vi "PicoScope5000aGetRapidBlockBulk.vi"(0 "error in":errorcluster, 5 "Device Info":T2, 7 "handle in":i16, 9 "enabled array":i16[](array[numeric]), 11 "Rapid Block Acquisition Settings":T1={"preTriggerSamples"=0, "postTriggerSamples"=1000, "timebase"=2, "Down-Sample Mode"=0, "Down Sample Ratio"=1, "Number of Captures"=10} {"Down Sample Ratio" min=1 step=1; "Down-Sample Mode" items=["None"=0, "Aggregate"=1, "Decimate"=2, "Average"=4]}) -> (2 "Channel A Buffer":i16[][](array[numeric]), 3 "Channel B Buffer":i16[][](array[numeric]), 4 "error out":errorcluster, 6 "handle out":i16, 8 "Port 0":i16[][](array[numeric]), 10 "Port 1":i16[][](array[numeric]), 12 "Num samples":u32, 13 "Channel C Buffer":i16[][](array[numeric]), 14 "Channel D Buffer":i16[][](array[numeric]))   [LabVIEW 2020]
doc: "This VI gets a set of blocks captured using rapid block mode. It outputs two-dimensional arrays for each channel that contain data from all the requested captures."
uses:
  ps5000a.dll
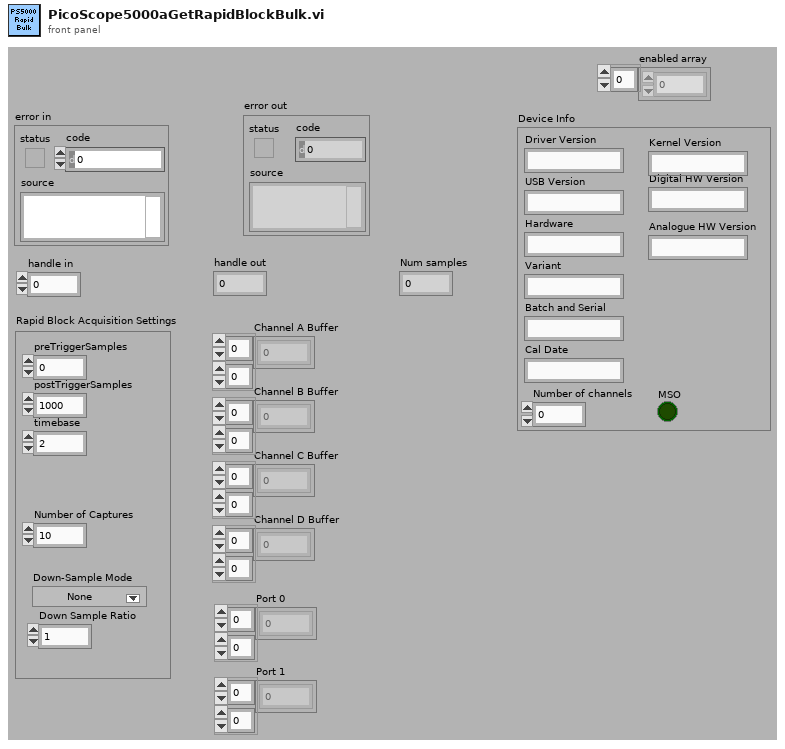
[diagram p1: front panel]
types:
  T1 = cluster{"preTriggerSamples":u32, "postTriggerSamples":u32, "timebase":u32, "Down-Sample Mode":i32, "Down Sample Ratio":u32, "Number of Captures":u32}
  T2 = cluster{"Driver Version":string, "USB Version":string, "Hardware":string, "Variant":string, "Batch and Serial":string, "Cal Date":string, "Kernel Version":string, "Digital HW Version":string, "Analogue HW Version":string, "MSO":bool, "Number of channels":i16}
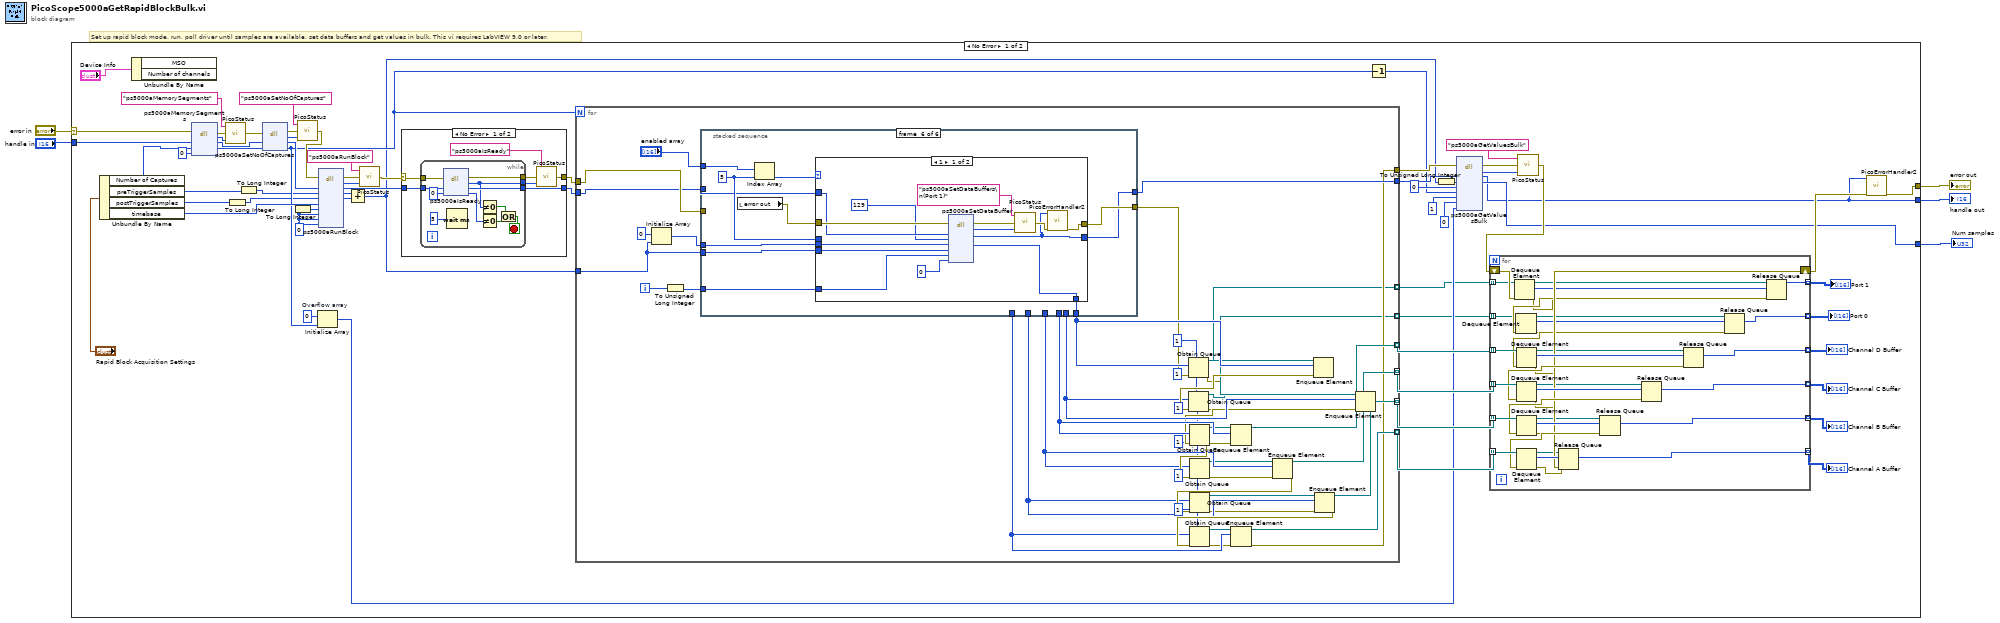
[diagram p0: block diagram]
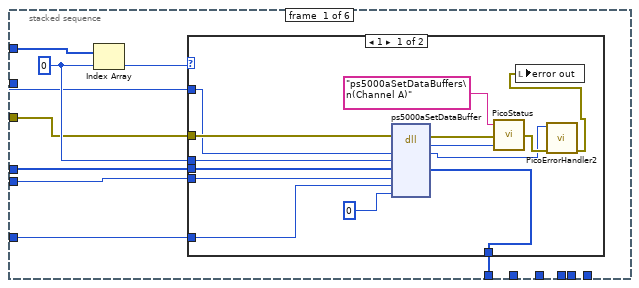
[diagram p2: hidden frame]
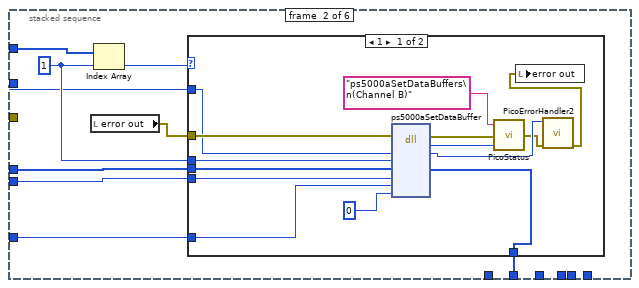
[diagram p4: hidden frame]
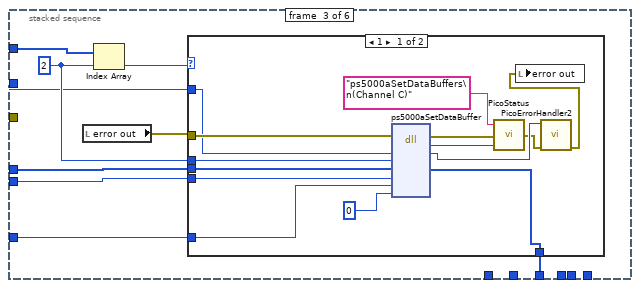
[diagram p6: hidden frame]
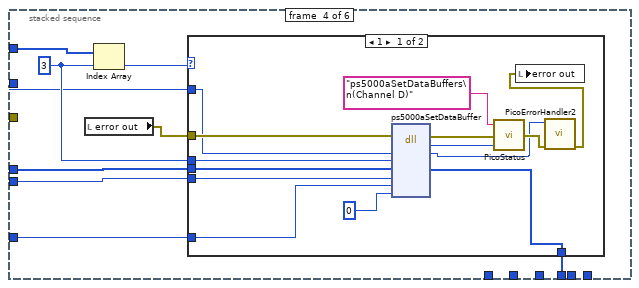
[diagram p8: hidden frame]
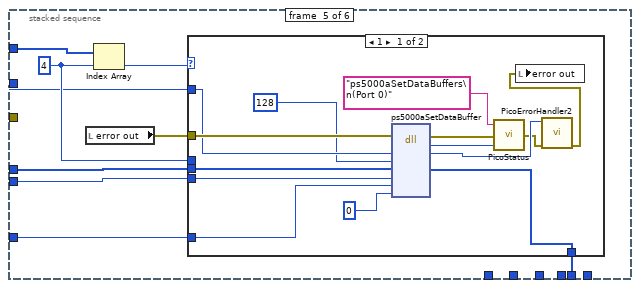
[diagram p10: hidden frame]
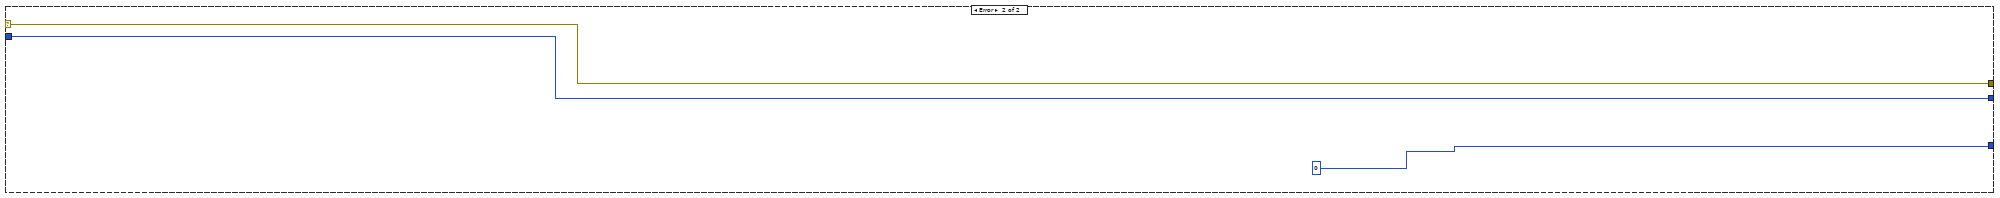
[diagram p14: hidden frame]
diagram:
  # "Set up rapid block mode, run, poll driver until samples are available, set data buffers and get values in bulk. This vi requires LabVIEW 9.0 or later."
  n1 = case shown="No Error" "error in" {
    selector: "error in" -> [w58 w311]
    tunnel: [w43 w311] -> w1
    tunnel: "handle in" -> [w57 w310]
    tunnel: [w15 w310] -> w3
    tunnel: [w19 0] -> w2
    frame No Error {
      w69 = u32 0 ("pParameter")
      n2 = Unbundle By Name("Rapid Block Acquisition Settings") -> ("Number of Captures"=w53:u32, "preTriggerSamples"=w13:u32, "postTriggerSamples"=w11:u32, "timebase"=w63:u32)
      n3 = Unbundle By Name("Device Info") -> ()  [unwired: 2 out]
      n4 = dll-call lib="ps5000a.dll" fn="ps5000aMemorySegments" ("ps3000.dll:_ps3000_open_unit@0")(error in=w58, "handle"=w57, "nSegments"=w53, "nMaxSamples"=0) -> (error out=w55:errorcluster, "PICO_STATUS"=w56:u32, "handle"=w50:i16, "nSegments"=w51:u32)  [unwired: 3 in, 1 out]
      n5 = call "PicoStatus.vi"("PICO STATUS"=w56, "error in"=w55, "source"="ps5000aMemorySegments") -> ("error out"=w49:errorcluster)
      n6 = To Long Integer(number=w11) -> (32bit integer=w10:i32)
      n7 = To Long Integer(number=w13) -> (32bit integer=w12:i32)
      n8 = dll-call lib="ps5000a.dll" fn="ps5000aSetNoOfCaptures" ("ps3000.dll:_ps3000_open_unit@0")(error in=w49, "handle"=w50, "nCaptures"=w51) -> (error out=w47:errorcluster, "PICO_STATUS"=w48:u32, "handle"=w44:i16, "nCaptures"=w21:u32)  [unwired: 2 in, 1 out]
      n9 = To Long Integer(number=w69) -> (32bit integer=w18:i32)
      n10 = call "PicoStatus.vi"("PICO STATUS"=w48, "error in"=w47, "source"="ps5000aSetNoOfCaptures") -> ("error out"=w45:errorcluster)
      n11 = Initialize Array "Overflow array"(i16 0 ("element"), w21) -> (w22:i16[])
      n12 = dll-call lib="ps5000a.dll" fn="ps5000aRunBlock" ("ps3000.dll:_ps3000_open_unit@0")(error in=w45, "handle"=w44, "preTriggerSamples"=w12, "postTriggerSamples"=w10, "timebase"=w63, "timeindisposedMs"=w18, "segmentIndex"=w69, "lpReady"=w69, "pParameter"=w69) -> (error out=w61:errorcluster, "PICO_STATUS"=w62:u32, "handle"=w68:i16, "preTriggerSamples"=w66:i32, "postTriggerSamples"=w65:i32)  [unwired: 7 in, 1 out]
      n13 = Add(x=w66, y=w65) -> (x+y=w20:i32)
      n14 = call "PicoStatus.vi"("PICO STATUS"=w62, "error in"=w61, "source"="ps5000aRunBlock") -> ("error out"=w60:errorcluster)
      n15 = case shown="No Error" w60 {
        selector: w60 -> [w293 w307]
        tunnel: w68 -> [w295 w308]
        tunnel: [w294 w308] -> w67
        tunnel: [w292 w307] -> w64
        frame No Error {
          n16 = while {
            tunnel: [w306] -> w294
            tunnel: w295 -> [w305]
            tunnel: [w300] -> w290
            tunnel: w293 -> [w299]
            tunnel: [w298] -> w291
            stop <- w304 stop-if-true
            n17 = dll-call lib="ps5000a.dll" fn="ps5000aIsReady" ("ps3000.dll:_ps3000_open_unit@0")(error in=w299, "handle"=w305, "ready"=i16 0) -> (error out=w298:errorcluster, "PICO_STATUS"=w300:u32, "handle"=w306:i16, "ready"=w301:i16)  [unwired: 2 in, 1 out]
            n18 = Wait (ms)(milliseconds to wait=u32 5 ("ready")) -> ()  [unwired: 1 out]
            n19 = Not Equal To 0?(x=w300) -> (x != 0?=w302:bool)
            n20 = Not Equal To 0?(x=w301) -> (x != 0?=w303:bool)
            n21 = Or(x=w302, y=w303) -> (x .or. y?=w304:bool)
          }
          n22 = call "PicoStatus.vi"("PICO STATUS"=w290, "error in"=w291, "source"="ps5000aIsReady") -> ("error out"=w292:errorcluster)
        }
        frame Error {
        }
      }
      n23 = for {
        N: w21 -> [_]
        tunnel: w67 -> [w134]
        tunnel: w64 -> [w135]
        tunnel: [w127] -> w33
        tunnel: [w143] -> w32 mode=indexing
        tunnel: [w142] -> w31 mode=indexing
        tunnel: [w141] -> w30 mode=indexing
        tunnel: [w140] -> w29 mode=indexing
        tunnel: [w133] -> w25
        tunnel: w20 -> [w136]
        tunnel: [w122] -> w9 mode=indexing
        tunnel: [w121] -> w8 mode=indexing
        i -> [w120]
        n24 = Initialize Array(i16 0 ("element"), w136) -> (w138:i16[])
        n25 = To Unsigned Long Integer(number=w120) -> (unsigned 32bit integer=w119:u32)
        n26 = stacked-sequence {
          tunnel: "enabled array" -> [w154 w177 w200 w223 w246 w271]
          tunnel: w135 -> [w152 _ _ _ _ _]
          tunnel: w134 -> [w151 w175 w198 w221 w244 w269]
          tunnel: w136 -> [w148 w174 w197 w220 w243 w268]
          tunnel: w138 -> [w147 w173 w196 w219 w242 w267]
          tunnel: [w150 _ _ _ _ _] -> w132
          tunnel: [_ _ _ _ _ w265] -> w124
          tunnel: [_ _ _ _ _ w264] -> w133
          tunnel: w119 -> [w149 w172 w195 w218 w241 w266]
          tunnel: [_ w171 _ _ _ _] -> w131
          tunnel: [_ _ w194 _ _ _] -> w130
          tunnel: [_ _ _ w217 _ _] -> w129
          tunnel: [_ _ _ _ w240 _] -> w126
          tunnel: [_ _ _ _ _ w262] -> w125
          frame #0 {
            w155 = 0 ("dimension size")
            n27 = Index Array(array=w154, index=w155) -> (element=w153:i16)
            n28 = case shown="1" w153 {
              tunnel: w155 -> [w166 _]
              tunnel: w152 -> [w168 _]
              tunnel: w151 -> [w167 _]
              tunnel: w148 -> [w164 _]
              tunnel: w147 -> [w165 _]
              tunnel: [w163 _] -> w150
              tunnel: w149 -> [w162 _]
              frame 1 {
                n29 = dll-call lib="ps5000a.dll" fn="ps5000aSetDataBuffer" ("ps3000.dll:_ps3000_open_unit@0")(error in=w168, "handle"=w167, "channel"=w166, "buffer"=w165, "bufferLth"=w164, "waveform"=w162, "downSampleRatioMode"=u32 0 ("segmentIndex")) -> (error out=w160:errorcluster, "PICO_STATUS"=w157:u32, "handle"=w156:i16, "buffer"=w163:i16[])  [unwired: 6 in, 1 out]
                n30 = call "PicoStatus.vi"("PICO STATUS"=w157, "error in"=w160, "source"="ps5000aSetDataBuffers\n(Channel A)") -> ("error out"=w159:errorcluster)
                n31 = call "PicoErrorHandler2.vi"("error in (no error)"=w159, "handle In"=w156) -> ("error out"=w158:errorcluster)  [unwired: 9 in]
                n32 = local write "error out"(w158) -> ()
              }
              frame 0, Default {
              }
            }
          }
          frame #1 {
            w178 = 1 ("dimension size")
            n33 = local read "error out"() -> (w170:errorcluster)
            n34 = Index Array(array=w177, index=w178) -> (element=w176:i16)
            n35 = case shown="1" w176 {
              tunnel: w178 -> [w189 _]
              tunnel: w170 -> [w191 _]
              tunnel: w175 -> [w190 _]
              tunnel: w174 -> [w187 _]
              tunnel: w173 -> [w188 _]
              tunnel: [w186 _] -> w171
              tunnel: w172 -> [w185 _]
              frame 1 {
                n36 = dll-call lib="ps5000a.dll" fn="ps5000aSetDataBuffer" ("ps3000.dll:_ps3000_open_unit@0")(error in=w191, "handle"=w190, "channel"=w189, "buffer"=w188, "bufferLth"=w187, "waveform"=w185, "downSampleRatioMode"=u32 0 ("segmentIndex")) -> (error out=w183:errorcluster, "PICO_STATUS"=w182:u32, "handle"=w180:i16, "buffer"=w186:i16[])  [unwired: 6 in, 1 out]
                n37 = call "PicoStatus.vi"("PICO STATUS"=w182, "error in"=w183, "source"="ps5000aSetDataBuffers\n(Channel B)") -> ("error out"=w179:errorcluster)
                n38 = call "PicoErrorHandler2.vi"("error in (no error)"=w179, "handle In"=w180) -> ("error out"=w181:errorcluster)  [unwired: 9 in]
                n39 = local write "error out"(w181) -> ()
              }
              frame 0, Default {
              }
            }
          }
          frame #2 {
            w201 = 2 ("dimension size")
            n40 = local read "error out"() -> (w193:errorcluster)
            n41 = Index Array(array=w200, index=w201) -> (element=w199:i16)
            n42 = case shown="1" w199 {
              tunnel: w201 -> [w212 _]
              tunnel: w193 -> [w214 _]
              tunnel: w198 -> [w213 _]
              tunnel: w197 -> [w210 _]
              tunnel: w196 -> [w211 _]
              tunnel: [w209 _] -> w194
              tunnel: w195 -> [w208 _]
              frame 1 {
                n43 = dll-call lib="ps5000a.dll" fn="ps5000aSetDataBuffer" ("ps3000.dll:_ps3000_open_unit@0")(error in=w214, "handle"=w213, "channel"=w212, "buffer"=w211, "bufferLth"=w210, "waveform"=w208, "downSampleRatioMode"=u32 0 ("segmentIndex")) -> (error out=w206:errorcluster, "PICO_STATUS"=w205:u32, "handle"=w204:i16, "buffer"=w209:i16[])  [unwired: 6 in, 1 out]
                n44 = call "PicoStatus.vi"("PICO STATUS"=w205, "error in"=w206, "source"="ps5000aSetDataBuffers\n(Channel C)") -> ("error out"=w203:errorcluster)
                n45 = call "PicoErrorHandler2.vi"("error in (no error)"=w203, "handle In"=w204) -> ("error out"=w202:errorcluster)  [unwired: 9 in]
                n46 = local write "error out"(w202) -> ()
              }
              frame 0, Default {
              }
            }
          }
          frame #3 {
            w224 = 3 ("dimension size")
            n47 = local read "error out"() -> (w216:errorcluster)
            n48 = Index Array(array=w223, index=w224) -> (element=w222:i16)
            n49 = case shown="1" w222 {
              tunnel: w224 -> [w235 _]
              tunnel: w216 -> [w237 _]
              tunnel: w221 -> [w236 _]
              tunnel: w220 -> [w233 _]
              tunnel: w219 -> [w234 _]
              tunnel: [w232 _] -> w217
              tunnel: w218 -> [w231 _]
              frame 1 {
                n50 = dll-call lib="ps5000a.dll" fn="ps5000aSetDataBuffer" ("ps3000.dll:_ps3000_open_unit@0")(error in=w237, "handle"=w236, "channel"=w235, "buffer"=w234, "bufferLth"=w233, "waveform"=w231, "downSampleRatioMode"=u32 0 ("segmentIndex")) -> (error out=w229:errorcluster, "PICO_STATUS"=w228:u32, "handle"=w225:i16, "buffer"=w232:i16[])  [unwired: 6 in, 1 out]
                n51 = call "PicoStatus.vi"("PICO STATUS"=w228, "error in"=w229, "source"="ps5000aSetDataBuffers\n(Channel D)") -> ("error out"=w226:errorcluster)
                n52 = call "PicoErrorHandler2.vi"("error in (no error)"=w226, "handle In"=w225) -> ("error out"=w227:errorcluster)  [unwired: 9 in]
                n53 = local write "error out"(w227) -> ()
              }
              frame 0, Default {
              }
            }
          }
          frame #4 {
            w247 = 4 ("dimension size")
            n54 = local read "error out"() -> (w239:errorcluster)
            n55 = Index Array(array=w246, index=w247) -> (element=w245:i16)
            n56 = case shown="1" w245 {
              tunnel: w247 -> [_ _]
              tunnel: w239 -> [w260 _]
              tunnel: w244 -> [w259 _]
              tunnel: w243 -> [w257 _]
              tunnel: w242 -> [w258 _]
              tunnel: [w256 _] -> w240
              tunnel: w241 -> [w255 _]
              frame 1 {
                n57 = dll-call lib="ps5000a.dll" fn="ps5000aSetDataBuffer" ("ps3000.dll:_ps3000_open_unit@0")(error in=w260, "handle"=w259, "channel"=u32 128, "buffer"=w258, "bufferLth"=w257, "waveform"=w255, "downSampleRatioMode"=u32 0 ("segmentIndex")) -> (error out=w253:errorcluster, "PICO_STATUS"=w252:u32, "handle"=w250:i16, "buffer"=w256:i16[])  [unwired: 6 in, 1 out]
                n58 = call "PicoStatus.vi"("PICO STATUS"=w252, "error in"=w253, "source"="ps5000aSetDataBuffers\n(Port 0)") -> ("error out"=w249:errorcluster)
                n59 = call "PicoErrorHandler2.vi"("error in (no error)"=w249, "handle In"=w250) -> ("error out"=w248:errorcluster)  [unwired: 9 in]
                n60 = local write "error out"(w248) -> ()
              }
              frame 0, Default {
              }
            }
          }
          frame #5 {
            w272 = 5 ("dimension size")
            n61 = local read "error out"() -> (w263:errorcluster)
            n62 = Index Array(array=w271, index=w272) -> (element=w270:i16)
            n63 = case shown="1" w270 {
              tunnel: w272 -> [_ _]
              tunnel: w263 -> [w285 w287]
              tunnel: w269 -> [w284 w288]
              tunnel: w268 -> [w282 _]
              tunnel: w267 -> [w283 _]
              tunnel: [w281 _] -> w262
              tunnel: w266 -> [w280 _]
              tunnel: [w275 w287] -> w265
              tunnel: [w273 w288] -> w264
              frame 1 {
                n64 = dll-call lib="ps5000a.dll" fn="ps5000aSetDataBuffer" ("ps3000.dll:_ps3000_open_unit@0")(error in=w285, "handle"=w284, "channel"=u32 129, "buffer"=w283, "bufferLth"=w282, "waveform"=w280, "downSampleRatioMode"=u32 0 ("segmentIndex")) -> (error out=w278:errorcluster, "PICO_STATUS"=w277:u32, "handle"=w273:i16, "buffer"=w281:i16[])  [unwired: 6 in, 1 out]
                n65 = call "PicoStatus.vi"("PICO STATUS"=w277, "error in"=w278, "source"="ps5000aSetDataBuffers\n(Port 1)") -> ("error out"=w274:errorcluster)
                n66 = call "PicoErrorHandler2.vi"("error in (no error)"=w274, "handle In"=w273) -> ("error out"=w275:errorcluster)  [unwired: 9 in]
              }
              frame 0, Default {
              }
            }
          }
        }
        n67 = Obtain Queue(max queue size (-1, unlimited)=1, element data type=w125, error in (no error)=w124) -> (queue out=w113:refnum<queue>, error out=w114:errorcluster)  [unwired: 2 in, 1 out]
        n68 = Enqueue Element(queue=w113, element=w125, error in (no error)=w114) -> (queue out=w121:refnum<queue>, error out=w128:errorcluster)  [unwired: 1 in, 1 out]
        n69 = Obtain Queue(max queue size (-1, unlimited)=1, element data type=w126, error in (no error)=w128) -> (queue out=w116:refnum<queue>, error out=w117:errorcluster)  [unwired: 2 in, 1 out]
        n70 = Enqueue Element(queue=w116, element=w126, error in (no error)=w117) -> (queue out=w122:refnum<queue>, error out=w123:errorcluster)  [unwired: 1 in, 1 out]
        n71 = Obtain Queue(max queue size (-1, unlimited)=1, element data type=w129, error in (no error)=w123) -> (queue out=w104:refnum<queue>, error out=w105:errorcluster)  [unwired: 2 in, 1 out]
        n72 = Enqueue Element(queue=w104, element=w129, error in (no error)=w105) -> (queue out=w143:refnum<queue>, error out=w146:errorcluster)  [unwired: 1 in, 1 out]
        n73 = Obtain Queue(max queue size (-1, unlimited)=1, element data type=w130, error in (no error)=w146) -> (queue out=w107:refnum<queue>, error out=w108:errorcluster)  [unwired: 2 in, 1 out]
        n74 = Enqueue Element(queue=w107, element=w130, error in (no error)=w108) -> (queue out=w142:refnum<queue>, error out=w145:errorcluster)  [unwired: 1 in, 1 out]
        n75 = Obtain Queue(max queue size (-1, unlimited)=1, element data type=w131, error in (no error)=w145) -> (queue out=w110:refnum<queue>, error out=w111:errorcluster)  [unwired: 2 in, 1 out]
        n76 = Enqueue Element(queue=w110, element=w131, error in (no error)=w111) -> (queue out=w141:refnum<queue>, error out=w144:errorcluster)  [unwired: 1 in, 1 out]
        n77 = Obtain Queue(max queue size (-1, unlimited)=1, element data type=w132, error in (no error)=w144) -> (queue out=w101:refnum<queue>, error out=w102:errorcluster)  [unwired: 2 in, 1 out]
        n78 = Enqueue Element(queue=w101, element=w132, error in (no error)=w102) -> (queue out=w140:refnum<queue>, error out=w127:errorcluster)  [unwired: 1 in, 1 out]
      }
      n79 = Decrement(x=w21) -> (x-1=w24:u32)
      n80 = To Unsigned Long Integer(number=w20) -> (unsigned 32bit integer=w17:u32)
      n81 = dll-call lib="ps5000a.dll" fn="ps5000aGetValuesBulk" ("ps3000.dll:_ps3000_open_unit@0")(error in=w33, "handle"=w25, "noOfSamples"=w17, "fromSegmentIndex"=u32 0, "toSegmentIndex"=w24, "downSampleRatio"=u32 1, "downSampleRatioMode"=u32 0, "overflow"=w22) -> (error out=w36:errorcluster, "PICO_STATUS"=w35:u32, "handle"=w15:i16, "noOfSamples"=w19:u32)  [unwired: 7 in, 1 out]
      n82 = call "PicoStatus.vi"("PICO STATUS"=w35, "error in"=w36, "source"="ps5000aGetValuesBulk") -> ("error out"=w34:errorcluster)
      n83 = for {
        tunnel: w29 -> [w100] mode=indexing
        tunnel: [w99] -> w37 mode=indexing
        shift-right: [w89] -> w41
        shift-left: w34 -> [w88]
        tunnel: w30 -> [w98] mode=indexing
        tunnel: w32 -> [w97] mode=indexing
        tunnel: w31 -> [w96] mode=indexing
        tunnel: [w92] -> w40 mode=indexing
        tunnel: [w91] -> w39 mode=indexing
        tunnel: [w90] -> w38 mode=indexing
        tunnel: w9 -> [w85] mode=indexing
        tunnel: w8 -> [w84] mode=indexing
        tunnel: [w83] -> w7 mode=indexing
        tunnel: [w82] -> w6 mode=indexing
        n84 = Dequeue Element(queue=w84, error in (no error)=w88) -> (queue out=w81:refnum<queue>, element=w82:i16[], error out=w80:errorcluster)  [unwired: 1 in, 1 out]
        n85 = Release Queue(queue=w81, error in (no error)=w80) -> (error out=w87:errorcluster)  [unwired: 1 in, 2 out]
        n86 = Dequeue Element(queue=w85, error in (no error)=w87) -> (queue out=w79:refnum<queue>, element=w83:i16[], error out=w78:errorcluster)  [unwired: 1 in, 1 out]
        n87 = Release Queue(queue=w79, error in (no error)=w78) -> (error out=w86:errorcluster)  [unwired: 1 in, 2 out]
        n88 = Dequeue Element(queue=w97, error in (no error)=w86) -> (queue out=w77:refnum<queue>, element=w92:i16[], error out=w76:errorcluster)  [unwired: 1 in, 1 out]
        n89 = Release Queue(queue=w77, error in (no error)=w76) -> (error out=w95:errorcluster)  [unwired: 1 in, 2 out]
        n90 = Dequeue Element(queue=w96, error in (no error)=w95) -> (queue out=w75:refnum<queue>, element=w91:i16[], error out=w74:errorcluster)  [unwired: 1 in, 1 out]
        n91 = Release Queue(queue=w75, error in (no error)=w74) -> (error out=w94:errorcluster)  [unwired: 1 in, 2 out]
        n92 = Dequeue Element(queue=w98, error in (no error)=w94) -> (queue out=w73:refnum<queue>, element=w90:i16[], error out=w72:errorcluster)  [unwired: 1 in, 1 out]
        n93 = Release Queue(queue=w73, error in (no error)=w72) -> (error out=w93:errorcluster)  [unwired: 1 in, 2 out]
        n94 = Dequeue Element(queue=w100, error in (no error)=w93) -> (queue out=w71:refnum<queue>, element=w99:i16[], error out=w70:errorcluster)  [unwired: 1 in, 1 out]
        n95 = Release Queue(queue=w71, error in (no error)=w70) -> (error out=w89:errorcluster)  [unwired: 1 in, 2 out]
      }
      "Channel D Buffer" <- w40
      "Channel C Buffer" <- w39
      "Channel B Buffer" <- w38
      "Channel A Buffer" <- w37
      "Port 0" <- w7
      "Port 1" <- w6
      n96 = call "PicoErrorHandler2.vi"("error in (no error)"=w41, "handle In"=w15) -> ("error out"=w43:errorcluster)  [unwired: 9 in]
    }
    frame Error {
    }
  }
  "handle out" <- w3
  "Num samples" <- w2
  "error out" <- w1
